vi "Bundle CMD Queue Cluster.vi"(10 "Message Data":variant, 11 "Message":string) -> (3 "Message Cluster":T1)   [LabVIEW 2020, in "Message Queue.lvlib"]
uses:
  Message Queue/Message Queue.lvlib
  Message Queue/Message Cluster.ctl
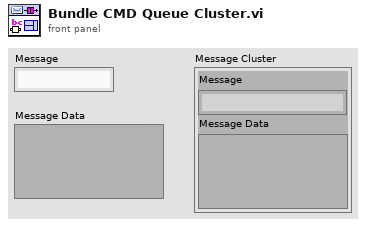
[diagram p1: front panel]
types:
  T1 = typedef "Message Queue.lvlib/Message Cluster.ctl" = cluster{"Message":string, "Message Data":variant}
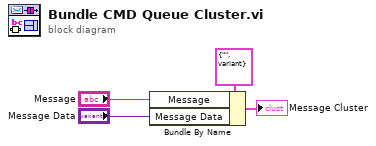
[diagram p0: block diagram]
diagram:
  n1 = Bundle By Name(cluster=T1 {"Message"="", "Message Data"=variant} ("Message Cluster"), "Message"="Message", "Message Data"="Message Data") -> (→"Message Cluster":T1)
